vi "Build Serial Cmd.vi"(6 "Display":string, 7 "Cmd":T1, 8 "error in (no error)":errorcluster, 9 "y":i64, 10 "x":i64, 11 "3010 in":refnum<class "3010.lvclass">) -> (0 "error out":errorcluster, 2 "Str Out":string, 3 "3010 out":refnum<class "3010.lvclass">)   [LabVIEW 2014, in "3010.lvclass"]
uses:
  3010.lvclass
  CPC.lvclass
  Controls/Enum Cmd.ctl
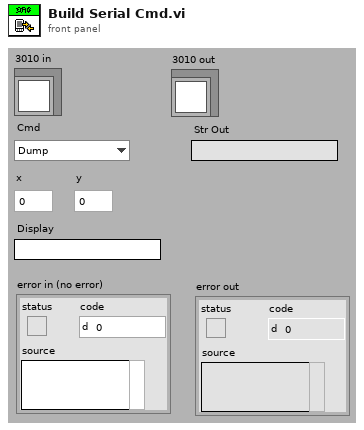
[diagram p1: front panel]
types:
  T1 = typedef "3010.lvclass/Enum Cmd.ctl" = enum16{"Dump", "Dump Cumulative", "Read Liquid Status", "Read Condenser Temperature", "Read Saturator Temperature", "Read Environment", "Read 6 s Buffer", "Read 1 s Buffer", "Read Concentration Display", "Read Delta T", "Read Vacuum Status", "Set Analog Voltage", "Execute Fill", "Clear Display Buffers"}
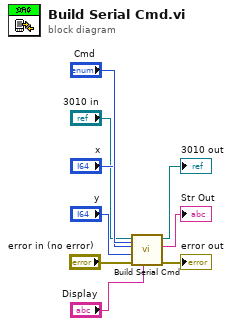
[diagram p0: block diagram]
diagram:
  n1 = call-parent "Build Serial Cmd.vi"("Display"="Display", "Cmd"="Cmd", "error in (no error)"="error in (no error)", "y"="y", "x"="x", "CPC in"="3010 in") -> ("error out"=→"error out":errorcluster, "Str Out"=→"Str Out":string, "CPC out"=→"3010 out":refnum<class "3010.lvclass">)  [unwired: 3 in]
